vi "写配置.vi"(5 "配置文件路径":path, 7 "枚举":enum16{"写", "读"}(ring), 10 "section":string, 11 "写入值":u32) -> (3 "读取值":u32)   [LabVIEW 2020]
uses:
  <vilib>/Utility/config.llb/Write Key (U32).vi
  <vilib>/Utility/config.llb/Read Key (U32).vi
  <vilib>/Utility/config.llb/NI_LVConfig.lvlib
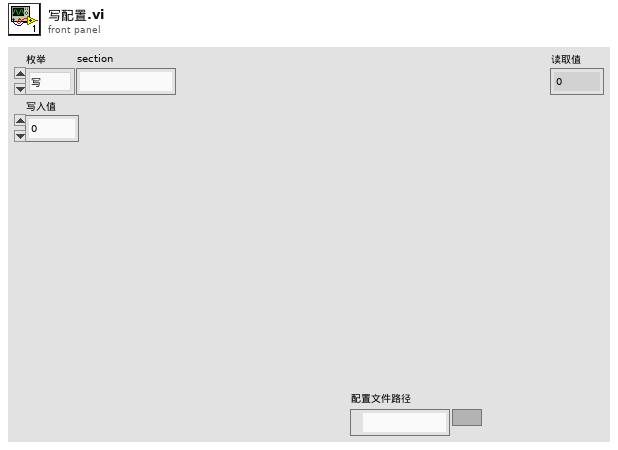
[diagram p1: front panel]
types:
  T1 = typedef "NI_LVConfig.lvlib/Config Data RefNum.ctl" = refnum<k1>
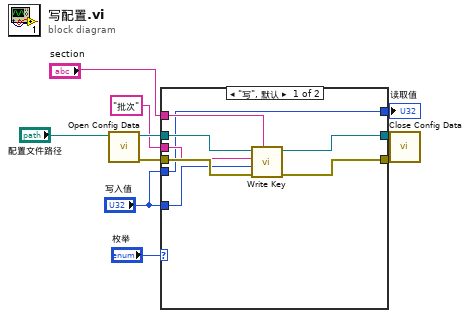
[diagram p0: block diagram]
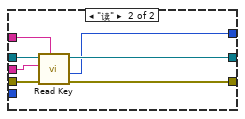
[diagram p2: hidden frame]
diagram:
  n1 = call <vilib>:"Open Config Data.vi"("configuration file path"="配置文件路径") -> ("error out"=w6:errorcluster, "refnum"=w9:T1)  [unwired: 8 in, 1 out]
  n2 = case shown="\"写\", 默认" "枚举" {
    tunnel: w9 -> [w18 w25]
    tunnel: [w17 w22] -> w8
    tunnel: w6 -> [w16 w24]
    tunnel: [w15 w23] -> w7
    tunnel: "写入值" -> [w12 _]
    tunnel: "section" -> [w14 w21]
    tunnel: "批次" ("key") -> [w13 w20]
    tunnel: [w11 w19] -> w3
    tunnel: "写入值" -> [w11 _]
    frame "写", Default {
      n3 = call-poly <vilib>:"Write Key.vi"("section"=w14, "error in (no error)"=w16, "value"=w12, "key"=w13, "refnum"=w18) -> ("error out"=w15:errorcluster, "refnum out"=w17:T1)  [unwired: 4 in, 1 out]
    }
    frame "读" {
      n4 = call-poly <vilib>:"Read Key.vi"("section"=w21, "error in (no error)"=w24, "key"=w20, "refnum"=w25) -> ("error out"=w23:errorcluster, "value"=w19:u32, "refnum out"=w22:T1)  [unwired: 4 in, 1 out]
    }
  }
  "读取值" <- w3
  n5 = call <vilib>:"Close Config Data.vi"("error in (no error)"=w7, "refnum"=w8) -> ()  [unwired: 8 in, 2 out]
